vi "_Parse Detected Allocation Segment.vi"(8 "error in (no error)":errorcluster, 10 "Input String":string, 11 "VISA resource name":refnum<visa-resource-name>) -> (0 "error out":errorcluster, 1 "Detected Allocation":T2, 2 "Reliability Results":T1, 3 "VISA resource name out":refnum<visa-resource-name>)   [LabVIEW 2020, in "Rohde&Schwarz CMWXP NR FR1 Measurement.lvlib"]
uses:
  <instrlib>/Rohde&Schwarz CMWXP NR FR1 Measurement/Rohde&Schwarz CMWXP NR FR1 Measurement.lvlib
  <instrlib>/Rohde&Schwarz CMWXP NR FR1 Measurement/Private/_SegReliability.ctl
  <instrlib>/Rohde&Schwarz CMWXP NR FR1 Measurement/Private/rsidr_core.llb/rsidr_core.lvlib
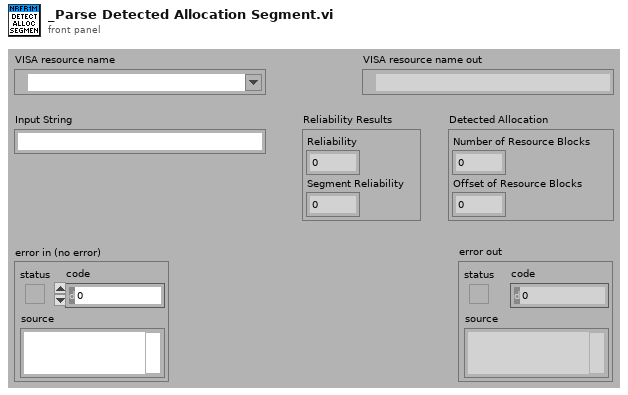
[diagram p1: front panel]
types:
  T1 = typedef "Rohde&Schwarz CMWXP NR FR1 Measurement.lvlib/_SegReliability.ctl" = cluster{"Reliability":i32, "Segment Reliability":i32}
  T2 = cluster{"Number of Resource Blocks":i32, "Offset of Resource Blocks":i32}
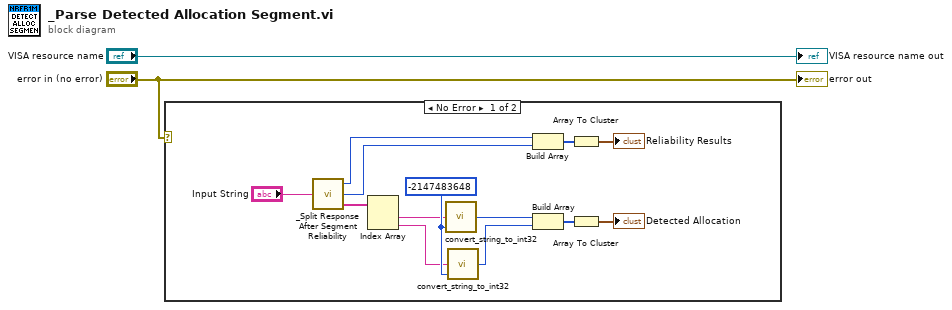
[diagram p0: block diagram]
diagram:
  n1 = case shown="No Error" "error in (no error)" {
    frame No Error {
      w15 = -2147483648
      n2 = call <instrlib>:"_Split Response After Segment Reliability.vi"("Input String"="Input String") -> ("Response out"=w14:string[], "Segment Reliability"=w9:i32, "Reliability"=w10:i32)
      n3 = Index Array(array=w14) -> (element #1=w12:string, element #2=w11:string)  [unwired: 2 in]
      n4 = call <instrlib>:"convert_string_to_int32.vi"("default (0)"=w15, "String in"=w12) -> ("int32 value out"=w5:i32)  [unwired: 3 in]
      n5 = call <instrlib>:"convert_string_to_int32.vi"("default (0)"=w15, "String in"=w11) -> ("int32 value out"=w4:i32)  [unwired: 3 in]
      n6 = Build Array(w10, w9) -> (w8:i32[])
      n7 = Build Array(w5, w4) -> (w6:i32[])
      n8 = Array To Cluster(array=w8) -> (cluster=→"Reliability Results":cluster{"[0]":i32, "[1]":i32})
      n9 = Array To Cluster(array=w6) -> (cluster=→"Detected Allocation":cluster{"[0]":i32, "[1]":i32})
    }
    frame Error {
    }
  }
  "VISA resource name out" <- "VISA resource name"
  "error out" <- "error in (no error)"
